vi "Voice_coil_camera_trigger.vi"() -> ()   [LabVIEW 2020]
uses:
  <vilib>/DAQmx/write.llb/DAQmx Write (Analog Wfm 1Chan NSamp).vi
  <vilib>/Utility/file.llb/Read Delimited Spreadsheet (DBL).vi
  <vilib>/DAQmx/create/channels.llb/DAQmx Create Channel (AO-Voltage-Basic).vi
  <vilib>/DAQmx/configure/timing.llb/DAQmx Timing (Sample Clock).vi
  <vilib>/DAQmx/miscellaneous.llb/DAQmx Fill In Error Info.vi
  <vilib>/DAQmx/create/channels.llb/DAQmx Create Channel (CO-Pulse Generation-Frequency).vi
  <vilib>/DAQmx/configure/timing.llb/DAQmx Timing (Implicit).vi
  <vilib>/DAQmx/create/channels.llb/DAQmx Create Channel (CO-Pulse Generation-Ticks).vi
  <resource>/objmgr/daqmx.rc
panel:
  in  "stop 2":bool caption="stop"
  in  "Delay between frames":dbl=25.0
  in  "Image acquisition time (ms)":dbl=1000.0
  in  "stop":bool
  in  "error in":errorcluster
  in  "File to read":path=path "C:/Users/lpk27/Documents/pan-ASLMsynched/pan-ASLM/Calibration files/newcalibration_voice coil input_25msflyback.txt"
  out "LabVIEW generated Sawtooth input (blue) and Camera trigger (red)":waveform(dbl)(graph)={"t0"=timestamp(0 s since 1904-01-01), "dt"=1.0, "Y"=array[3075 elements]}
  out "# Samples written per channel":u32=3075
  out "actual frequency":dbl=1000.0
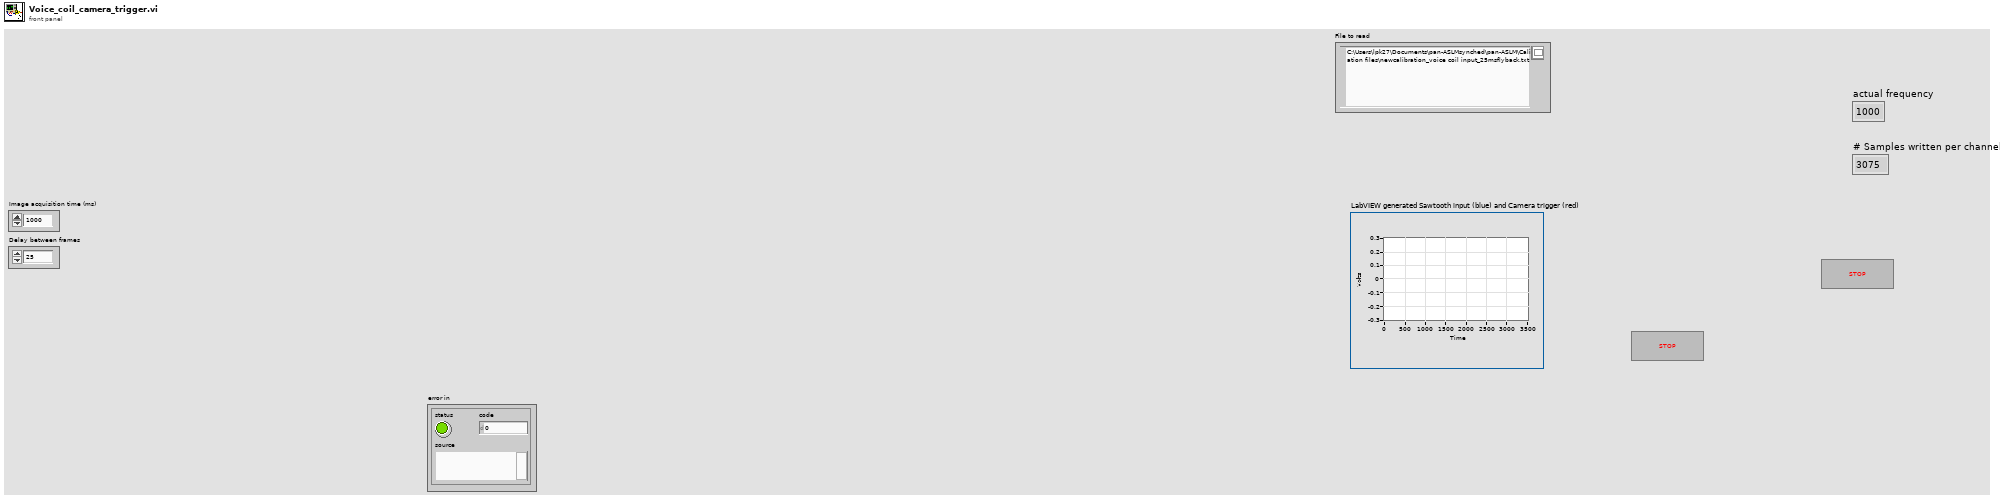
[diagram p1: front panel]
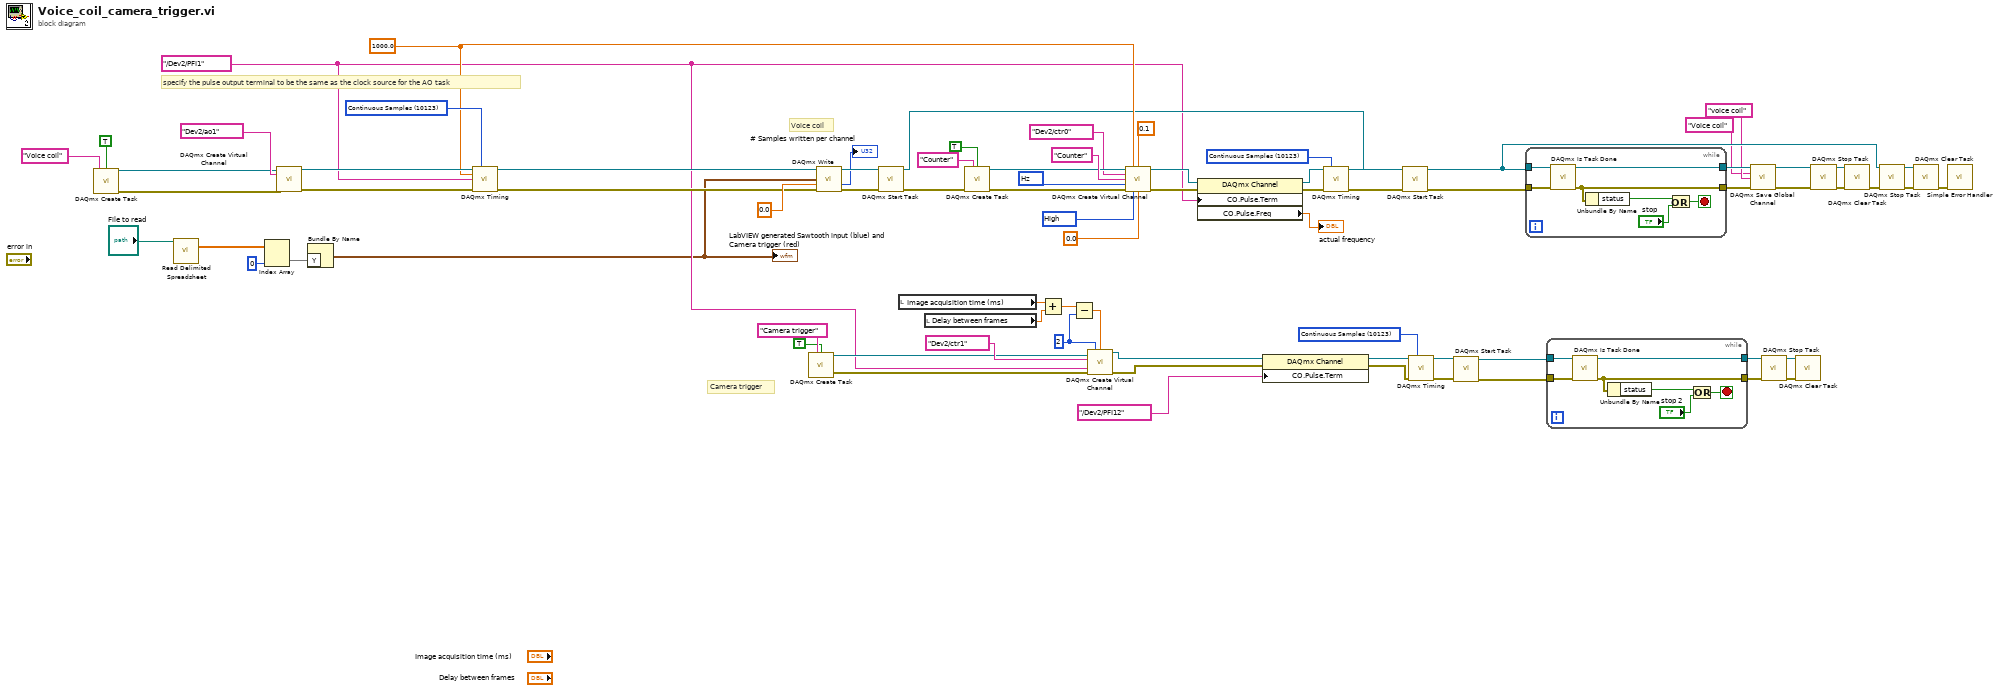
[diagram p0: block diagram]
diagram:
  w20 = u32 2 ("high ticks")
  w30 = 10123 items=["Finite Samples"=10178, "Continuous Samples"=10123, "Hardware Timed Single Point"=12522] ("sample mode")
  w57 = 10192 items=["High"=10192, "Low"=10214] ("idle state")
  w58 = 10373 items=["Hz"=10373] ("units")
  w14 = tag "/Dev2/PFI1" ("CO.Pulse.Term")
  w51 = 10123 items=["Finite Samples"=10178, "Continuous Samples"=10123, "Hardware Timed Single Point"=12522] ("sample mode")
  w50 = 1000.0 ("rate")
  w76 = 10123 items=["Finite Samples"=10178, "Continuous Samples"=10123, "Hardware Timed Single Point"=12522] ("sample mode")
  # "Camera trigger"
  # "Voice coil"
  # "specify the pulse output terminal to be the same as the clock source for the AO task"
  n1 = call <vilib>:"DAQmx Create Task.vi"("new task name"="Voice coil", "auto cleanup"=TRUE) -> ("task out"=w44:refnum<k21>, "error out"=w43:errorcluster)  [unwired: 12 in]
  n2 = call-poly <vilib>:"Read Delimited Spreadsheet.vi"("file path (dialog if empty)"="File to read") -> ("all rows"=w48:dbl[][])  [unwired: 9 in, 5 out]
  n3 = Index Array(array=w48, index (col)=0 ("disabled index (col)")) -> (element=w46:dbl[])  [unwired: 1 in]
  n4 = call-poly <vilib>:"DAQmx Create Virtual Channel.vi"("task in"=w44, "physical channels"=tag "Dev2/ao1", "error in"=w43) -> ("task out"=w78:refnum<k21>, "error out"=w77:errorcluster)  [unwired: 11 in]
  n5 = Bundle By Name("Y"=w46) -> (w7:waveform(dbl))  [unwired: 1 in]
  "LabVIEW generated Sawtooth input (blue) and Camera trigger (red)" <- w7
  n6 = call-poly <vilib>:"DAQmx Timing.vi"("task/channels in"=w78, "sample mode"=w76, "rate"=w50, "source"=w14, "error in"=w77) -> ("task out"=w53:refnum<k21>, "error out"=w52:errorcluster)  [unwired: 9 in]
  n7 = call <vilib>:"DAQmx Create Task.vi"("new task name"="Camera trigger", "auto cleanup"=TRUE) -> ("task out"=w16:refnum<k21>, "error out"=w17:errorcluster)  [unwired: 12 in]
  n8 = call-poly <vilib>:"DAQmx Write.vi"("task/channels in"=w53, "data"=w7, "timeout"=0.0, "error in"=w52) -> ("task out"=w63:refnum<k21>, "number of samples written per channel"=→"# Samples written per channel":u32, "error out"=w62:errorcluster)  [unwired: 9 in]
  n9 = call <vilib>:"DAQmx Start Task.vi"("task/channels in"=w63, "error in"=w62) -> ("task out"=w33:refnum<k21>, "error out"=w56:errorcluster)  [unwired: 12 in]
  n10 = local read "Image acquisition time (ms)"() -> (w23:dbl)
  n11 = local read "Delay between frames"() -> (w22:dbl)
  n12 = call <vilib>:"DAQmx Create Task.vi"("new task name"="Counter", "auto cleanup"=TRUE, "error in"=w56) -> ("task out"=w71:refnum<k21>, "error out"=w69:errorcluster)  [unwired: 11 in]
  n13 = Add(x=w23, y=w22) -> (x+y=w21:dbl)
  n14 = Subtract(x=w21, y=w20) -> (x-y=w19:dbl)
  n15 = call-poly <vilib>:"DAQmx Create Virtual Channel.vi"("task in"=w16, "high ticks"=w20, "low ticks"=w19, "counter"=tag "Dev2/ctr1", "source of ticks"=w14, "error in"=w17) -> ("task out"=w32:refnum<k21>, "error out"=w27:errorcluster)  [unwired: 8 in]
  n16 = call-poly <vilib>:"DAQmx Create Virtual Channel.vi"("task in"=w71, "frequency"=w50, "duty cycle"=0.1, "counter"=tag "Dev2/ctr0", "name to assign"="Counter", "units"=w58, "error in"=w69, "idle state"=w57, "initial delay"=0.0) -> ("task out"=w68:refnum<k21>, "error out"=w67:errorcluster)  [unwired: 5 in]
  n17 = property class="DAQmx Channel"(reference=w68, error in=w67, "CO.Pulse.Term"=w14) -> (reference out=w64:refnum<k21>, error out=w65:errorcluster, "CO.Pulse.Freq"=→"actual frequency":dbl)
  n18 = property class="DAQmx Channel"(reference=w32, error in=w27, "CO.Pulse.Term"=tag "/Dev2/PFI12") -> (reference out=w25:refnum<k21>, error out=w31:errorcluster)
  n19 = call-poly <vilib>:"DAQmx Timing.vi"("task/channels in"=w64, "sample mode"=w51, "error in"=w65) -> ("task out"=w74:refnum<k21>, "error out"=w73:errorcluster)  [unwired: 11 in]
  n20 = call <vilib>:"DAQmx Start Task.vi"("task/channels in"=w74, "error in"=w73) -> ("error out"=w34:errorcluster)  [unwired: 12 in, 1 out]
  n21 = call-poly <vilib>:"DAQmx Timing.vi"("task/channels in"=w25, "sample mode"=w30, "error in"=w31) -> ("task out"=w29:refnum<k21>, "error out"=w28:errorcluster)  [unwired: 11 in]
  n22 = call <vilib>:"DAQmx Start Task.vi"("task/channels in"=w29, "error in"=w28) -> ("task out"=w9:refnum<k21>, "error out"=w8:errorcluster)  [unwired: 12 in]
  n23 = while {
    tunnel: w33 -> [w85]
    tunnel: w34 -> [w84]
    tunnel: [w83] -> w6
    tunnel: [w82] -> w5
    stop <- w79 stop-if-true
    n24 = call <vilib>:"DAQmx Is Task Done.vi"("task/channels in"=w85, "error in"=w84) -> ("task out"=w83:refnum<k21>, "error out"=w82:errorcluster)  [unwired: 11 in, 1 out]
    n25 = Unbundle By Name(w82) -> ("status"=w81:bool)
    n26 = Or(x=w81, y="stop") -> (x .or. y?=w79:bool)
  }
  n27 = while {
    tunnel: w9 -> [w92]
    tunnel: w8 -> [w91]
    tunnel: [w90] -> w12
    tunnel: [w89] -> w13
    stop <- w86 stop-if-true
    n28 = call <vilib>:"DAQmx Is Task Done.vi"("task/channels in"=w92, "error in"=w91) -> ("task out"=w90:refnum<k21>, "error out"=w89:errorcluster)  [unwired: 11 in, 1 out]
    n29 = Unbundle By Name(w89) -> ("status"=w88:bool)
    n30 = Or(x=w88, y="stop 2") -> (x .or. y?=w86:bool)
  }
  n31 = call <vilib>:"DAQmx Save Global Channel.vi"("task/channels in"=w6, "channel name"="Voice coil", "save as"="voice coil", "error in"=w5) -> ("task out"=w3:refnum<k21>, "error out"=w4:errorcluster)  [unwired: 10 in]
  n32 = call <vilib>:"DAQmx Stop Task.vi"("task/channels in"=w12, "error in"=w13) -> ("task out"=w11:refnum<k21>, "error out"=w10:errorcluster)  [unwired: 12 in]
  n33 = call <vilib>:"DAQmx Clear Task.vi"("task in"=w11, "error in"=w10) -> ()  [unwired: 13 in, 1 out]
  n34 = call <vilib>:"DAQmx Stop Task.vi"("task/channels in"=w3, "error in"=w4) -> ("task out"=w38:refnum<k21>, "error out"=w37:errorcluster)  [unwired: 12 in]
  n35 = call <vilib>:"DAQmx Clear Task.vi"("task in"=w38, "error in"=w37) -> ("error out"=w36:errorcluster)  [unwired: 13 in]
  n36 = call <vilib>:"DAQmx Stop Task.vi"("task/channels in"=w33, "error in"=w36) -> ("task out"=w39:refnum<k21>, "error out"=w40:errorcluster)  [unwired: 12 in]
  n37 = call <vilib>:"DAQmx Clear Task.vi"("task in"=w39, "error in"=w40) -> ("error out"=w35:errorcluster)  [unwired: 13 in]
  n38 = call <vilib>:"Simple Error Handler.vi"("error in (no error)"=w35) -> ()  [unwired: 4 in, 5 out]
